vi "Read registry info.vi"(10 "settings directory in":path, 11 "change directory":bool) -> (0 "settings directory":path)   [LabVIEW 2014]
uses:
  <vilib>/registry/registry.llb/Registry RtKey.ctl
  <vilib>/registry/registry.llb/Registry SAM.ctl
  <vilib>/registry/registry.llb/Read Registry Value Simple STR.vi
  Instance           1 26Saved   Read registry info .vi
  <vilib>/registry/registry.llb/Write Registry Value Simple STR.vi
  Instance           3 26Saved   Read registry info .vi
  Instance           2 26Saved   Read registry info .vi
panel:
  out "String/Binary data":string
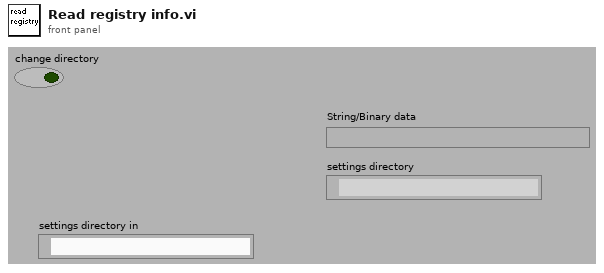
[diagram p1: front panel]
types:
  T1 = typedef "Registry RtKey.ctl" = enum32{"HKEY_CLASSES_ROOT", "HKEY_CURRENT_USER", "HKEY_LOCAL_MACHINE", "HKEY_USERS", "HKEY_PERFORMANCE_DATA", "HKEY_CURRENT_CONFIG", "HKEY_DYN_DATA"}
  T2 = typedef "Registry refnum.ctl" = refnum<k1>
  T3 = enum32{"REG_OPTION_NON_VOLATILE", "REG_OPTION_VOLATILE", "REG_OPTION_BACKUP_RESTORE"}
  T4 = typedef "Registry SAM.ctl" = enum32{"KEY_QUERY_VALUE", "KEY_SET_VALUE", "KEY_CREATE_SUB_KEY", "KEY_ENUMERATE_SUB_KEYS", "KEY_NOTIFY", "KEY_CREATE_LINK", "KEY_READ", "KEY_WRITE", "KEY_ALL_ACCESS", "KEY_READ | KEY_WRITE"}
  T5 = enum16{"Left Button", "Center Button", "Right Button", "Window Close"}
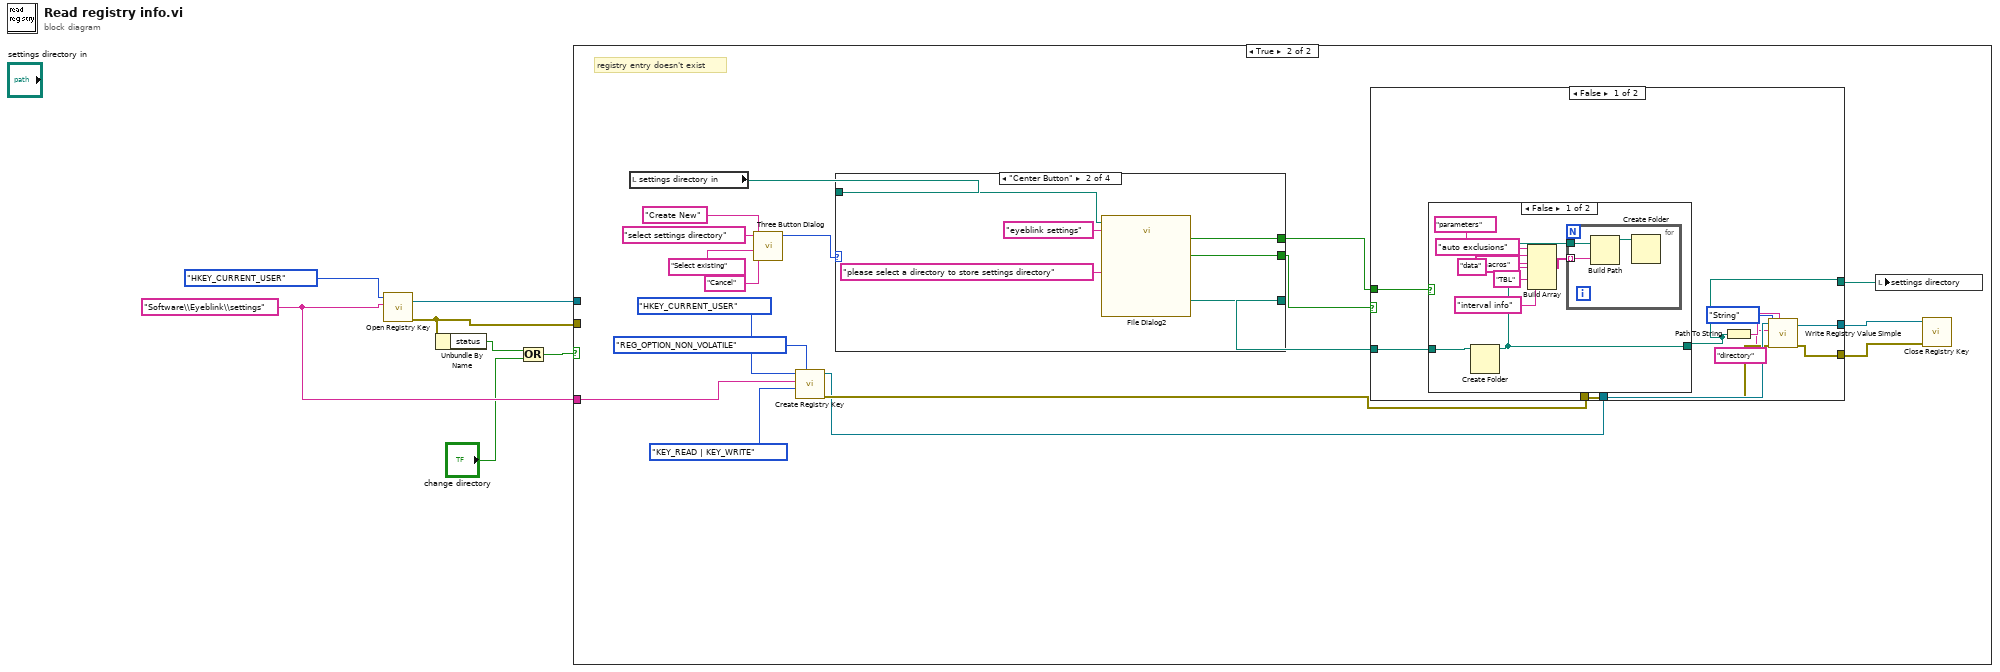
[diagram p0: block diagram]
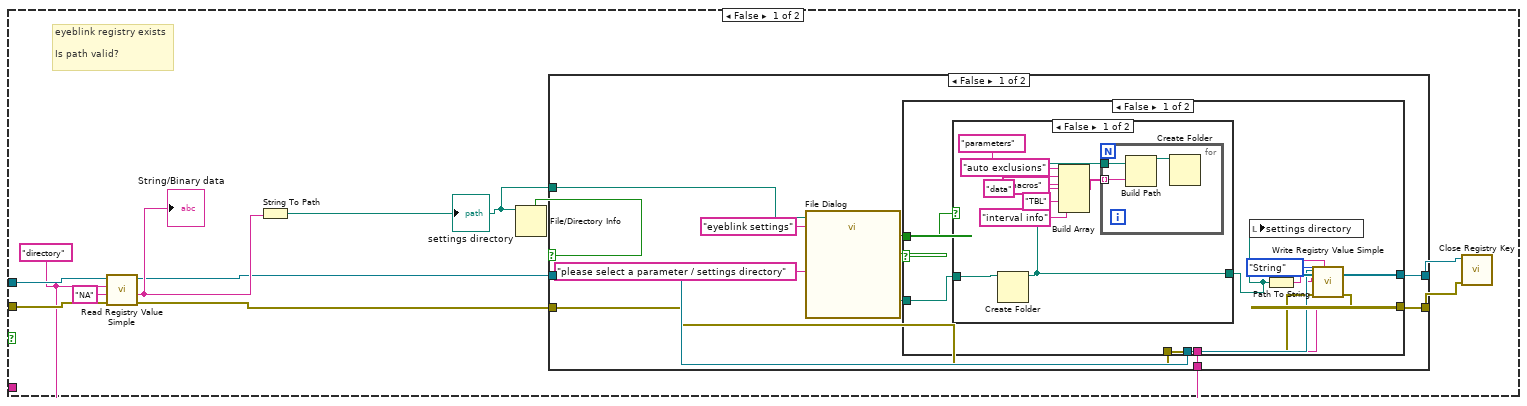
[diagram p2: hidden frame]
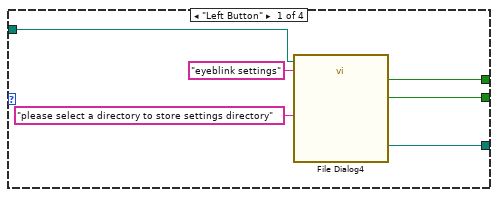
[diagram p6: hidden frame]
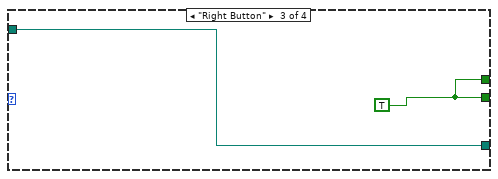
[diagram p7: hidden frame]
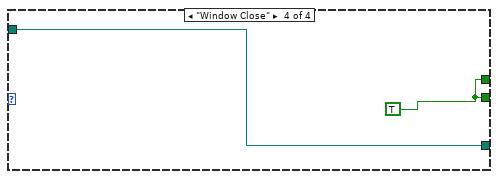
[diagram p8: hidden frame]
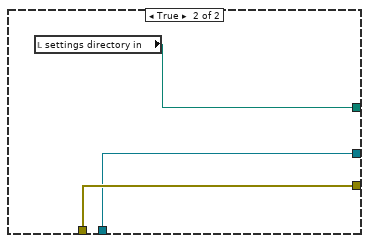
[diagram p10: hidden frame]
diagram:
  w4 = "Software\\Eyeblink\\settings" ("subkey")
  n1 = call <vilib>:"Open Registry Key.vi"("subkey"=w4, "root key (HKEY_LOCAL_MACHINE)"=Registry_RtKey."HKEY_CURRENT_USER") -> ("error out"=w5:errorcluster, "refnum out"=w6:T2)  [unwired: 8 in]
  n2 = Unbundle By Name(w5) -> ("status"=w2:bool)
  n3 = Or(x=w2, y="change directory") -> (x .or. y?=w3:bool)
  n4 = case shown="True" w3 {
    tunnel: w6 -> [w18 _]
    tunnel: w5 -> [w17 _]
    tunnel: w4 -> [_ w73]
    frame False {
      w8 = "directory" ("value")
      # "eyeblink registry exists\n\nIs path valid?"
      n5 = call-poly <vilib>:"Read Registry Value Simple.vi"("error in (no error)"=w17, "default data"="NA", "value"=w8, "refnum"=w18) -> ("error out"=w11:errorcluster, "String/Binary data"=w15:string, "refnum out"=w13:T2)  [unwired: 2 in, 1 out]
      "String/Binary data" <- w15
      n6 = String To Path(string=w15) -> (path=w9:path)
      "settings directory" <- w9
      n7 = File/Directory Info(path=w9) -> (directory=w10:bool)  [unwired: 1 in, 6 out]
      n8 = case shown="False" w10 {
        tunnel: [w23 w56] -> w14
        tunnel: w13 -> [w21 w56]
        tunnel: [w22 w55] -> w12
        tunnel: w11 -> [w20 w55]
        tunnel: w9 -> [w29 _]
        tunnel: w8 -> [w19 _]
        frame False {
          n9 = call "File Dialog"("start path"=w29, "prompt"="please select a parameter / settings directory", "default name"="eyeblink settings") -> ("selected path"=w24:path, "exists"=w25:bool, "cancelled"=w26:bool)  [unwired: 9 in, 1 out]
          n10 = case shown="False" w26 {
            tunnel: w25 -> [w30 _]
            tunnel: w24 -> [w31 _]
            tunnel: [w39 w53] -> w23
            tunnel: [w38 w54] -> w22
            tunnel: w21 -> [w37 w53]
            tunnel: w20 -> [w36 w54]
            tunnel: w19 -> [w34 _]
            frame False {
              n11 = case shown="False" w30 {
                tunnel: w31 -> [w48 w52]
                tunnel: [w47 w52] -> w32
                frame False {
                  n12 = Create Folder(path (use dialog)=w48) -> (created path=w47:path)  [unwired: 2 in, 2 out]
                  n13 = Build Array("parameters" ("name or relative path"), "auto exclusions" ("name or relative path"), "macros" ("name or relative path"), "data" ("element"), "TBL" ("element"), "interval info" ("element")) -> (w44:string[])
                  n14 = for {
                    tunnel: w44 -> [w51] mode=indexing
                    tunnel: w47 -> [w50]
                    n15 = Build Path(base path=w50, name or relative path=w51) -> (appended path=w49:path)
                    n16 = Create Folder(path (use dialog)=w49) -> ()  [unwired: 2 in, 3 out]
                  }
                }
                frame True {
                }
              }
              n17 = local write "settings directory"(w32) -> ()
              n18 = Path To String(path=w32) -> (string=w35:string)
              n19 = call-poly <vilib>:"Write Registry Value Simple.vi"("String/Binary data"=w35, "error in (no error)"=w36, "simple data type"=enum16{"String", "Binary", "DWORD"}."String", "value"=w34, "refnum"=w37) -> ("error out"=w38:errorcluster, "refnum out"=w39:T2)  [unwired: 3 in]
            }
            frame True {
            }
          }
        }
        frame True {
        }
      }
      n20 = call <vilib>:"Close Registry Key.vi"("error in (no error)"=w12, "refnum"=w14) -> ()  [unwired: 5 in, 1 out]
    }
    frame True {
      # "registry entry doesn't exist"
      n21 = local read "settings directory in"() -> (w62:path)
      n22 = call <vilib>:"Three Button Dialog.vi"("Right Button Text (\"Cancel\")"="Cancel" ("Right Button Text (\"Cancel\")"), "Center Button Text (\"No\")"="Select existing" ("Right Button Text (\"Cancel\")"), "Left Button Text (\"Yes\")"="Create New" ("Left Button Text (\"Yes\")"), "message"="select settings directory") -> ("Which Button?"=w57:T5)  [unwired: 7 in]
      n23 = call <vilib>:"Create Registry Key.vi"("options"=T3."REG_OPTION_NON_VOLATILE", "security access mask (KEY_READ | KEY_WRITE)"=Registry_SAM."KEY_READ | KEY_WRITE", "subkey"=w73, "root key (HKEY_LOCAL_MACHINE)"=Registry_RtKey."HKEY_CURRENT_USER") -> ("error out"=w67:errorcluster, "refnum out"=w66:T2)  [unwired: 5 in, 1 out]
      n24 = case shown="\"Center Button\"" w57 {
        tunnel: [w78 w84 w87 w90] -> w70
        tunnel: [w77 w83 w87 w90] -> w69
        tunnel: [w76 w82 w88 w89] -> w68
        tunnel: w62 -> [w75 w81 w88 w89]
        frame "Left Button" {
          n25 = call "File Dialog4"("start path"=w75, "prompt"="please select a directory to store settings directory", "default name"="eyeblink settings") -> ("selected path"=w76:path, "exists"=w77:bool, "cancelled"=w78:bool)  [unwired: 9 in, 1 out]
        }
        frame "Center Button" {
          n26 = call "File Dialog2"("start path"=w81, "prompt"="please select a directory to store settings directory", "default name"="eyeblink settings") -> ("selected path"=w82:path, "exists"=w83:bool, "cancelled"=w84:bool)  [unwired: 9 in, 1 out]
        }
        frame "Right Button" {
          w87 = TRUE ("cancelled")
        }
        frame "Window Close" {
          w90 = TRUE ("cancelled")
        }
      }
      n27 = case shown="False" w70 {
        tunnel: w69 -> [w100 _]
        tunnel: w68 -> [w99 _]
        tunnel: [w98 w115] -> w65
        tunnel: [w97 w116] -> w64
        tunnel: w66 -> [w96 w115]
        tunnel: w67 -> [w95 w116]
        tunnel: [w94 w114] -> w63
        frame False {
          n28 = case shown="False" w100 {
            tunnel: w99 -> [w109 w113]
            tunnel: [w108 w113] -> w94
            frame False {
              n29 = Create Folder(path (use dialog)=w109) -> (created path=w108:path)  [unwired: 2 in, 2 out]
              n30 = Build Array("parameters" ("name or relative path"), "auto exclusions" ("name or relative path"), "macros" ("name or relative path"), "data" ("element"), "TBL" ("element"), "interval info" ("element")) -> (w105:string[])
              n31 = for {
                tunnel: w105 -> [w112] mode=indexing
                tunnel: w108 -> [w111]
                n32 = Build Path(base path=w111, name or relative path=w112) -> (appended path=w110:path)
                n33 = Create Folder(path (use dialog)=w110) -> ()  [unwired: 2 in, 3 out]
              }
            }
            frame True {
            }
          }
          n34 = Path To String(path=w94) -> (string=w93:string)
          n35 = call-poly <vilib>:"Write Registry Value Simple.vi"("String/Binary data"=w93, "error in (no error)"=w95, "simple data type"=enum16{"String", "Binary", "DWORD"}."String", "value"="directory", "refnum"=w96) -> ("error out"=w97:errorcluster, "refnum out"=w98:T2)  [unwired: 3 in]
        }
        frame True {
          n36 = local read "settings directory in"() -> (w114:path)
        }
      }
      n37 = local write "settings directory"(w63) -> ()
      n38 = call <vilib>:"Close Registry Key.vi"("error in (no error)"=w64, "refnum"=w65) -> ()  [unwired: 5 in, 1 out]
    }
  }
